vi "Create DTC Section.vi"(8 "error in (no error)":errorcluster, 10 "Name":string, 11 "Item Ref in":T1 format="%.0x") -> (0 "error out":errorcluster)   [LabVIEW 2019, in "J1939 Addon Shared.lvlib"]
uses:
  J1939 Addon Shared.lvlib
  Constants.vi
  <vilib>/NI VeriStand/Custom Device API/Custom Device Channel Type.ctl
  <vilib>/NI VeriStand/Custom Device API/Custom Device API.lvlib
  <vilib>/NI VeriStand/Custom Device API/Custom Device Channel.ctl
  <vilib>/NI/NI VeriStand Advanced SysDef API/SysDef API/Advanced System Definition.lvlib
  <vilib>/NI VeriStand/Custom Device API/Custom Device Item Ref.ctl
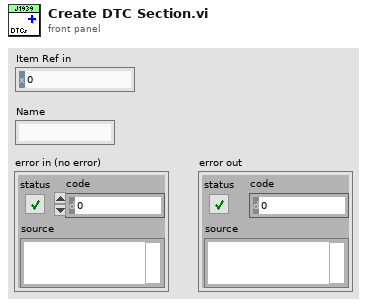
[diagram p1: front panel]
types:
  T1 = typedef "Custom Device API.lvlib/Custom Device Item Ref.ctl" = u64
  T2 = typedef "Custom Device API.lvlib/Custom Device Channel.ctl" = cluster{"Type":T3, "Units":string, "Default Value":dbl, "Faultable":bool, "Scalable":bool}
  T3 = typedef "Custom Device API.lvlib/Custom Device Channel Type.ctl" = enum16{"Input", "Output"}
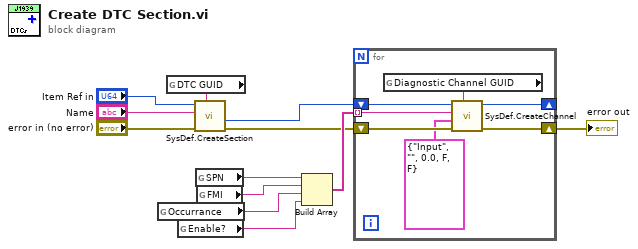
[diagram p0: block diagram]
diagram:
  n1 = global read "Constants.vi" "Occurrance"() -> (w9:string)
  n2 = global read "Constants.vi" "DTC GUID"() -> (w1:string)
  n3 = global read "Constants.vi" "Enable?"() -> (w11:string)
  n4 = call <vilib>:"SysDef.CreateSection.vi"("GUID"=w1, "error in (no error)"="error in (no error)", "Name"="Name", "nodeID"="Item Ref in") -> ("error out"=w5:errorcluster, "New NodeID"=w6:u64)  [unwired: 4 in, 2 out]
  n5 = global read "Constants.vi" "SPN"() -> (w7:string)
  n6 = global read "Constants.vi" "FMI"() -> (w8:string)
  n7 = Build Array(w7, w8, w9, w11) -> (w10:string[])
  n8 = for {
    tunnel: w10 -> [w16] mode=indexing
    shift-right: [w14] -> w12
    shift-left: w5 -> [w19]
    shift-right: [w13] -> _
    shift-left: w6 -> [w18]
    n9 = global read "Constants.vi" "Diagnostic Channel GUID"() -> (w17:string)
    n10 = call <vilib>:"SysDef.CreateChannel.vi"("GUID"=w17, "error in (no error)"=w19, "Channel"=T2 {"Type"=enum."Input", "Units"="", "Default Value"=0.0, "Faultable"=FALSE, "Scalable"=FALSE}, "Name"=w16, "nodeID"=w18) -> ("error out"=w14:errorcluster, "nodeID out"=w13:u64)  [unwired: 3 in, 2 out]
  }
  "error out" <- w12
